vi "Get Devs and Channels.vi"(8 "error in (no error)":errorcluster, 11 "Simulated Sequencer in":refnum<class "Simulated Sequencer.lvclass">) -> (0 "error out":errorcluster, 3 "Simulated Sequencer out":refnum<class "Simulated Sequencer.lvclass">)   [LabVIEW 2015, in "Simulated Sequencer.lvlib" / "Simulated Sequencer.lvclass"]
uses:
  Simulated Sequencer.lvclass
  Sequencer/Sequencer/Daq Channel Info.ctl
  Sequencer/Sequencer/Sequencer.lvclass
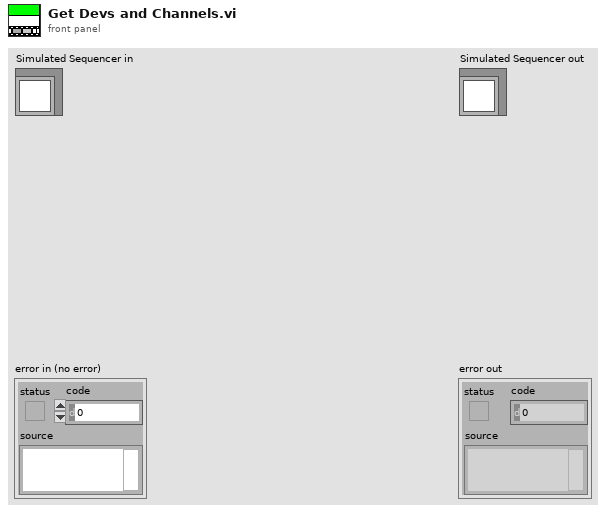
[diagram p1: front panel]
types:
  T1 = typedef "Sequencer.lvlib/Sequencer.lvclass/Daq Channel Info.ctl" = cluster{"DevNames":tag[], "AO.PhysicalChans":tag[][], "DO.Lines":tag[][], "AI.PhysicalChans":tag[][]}
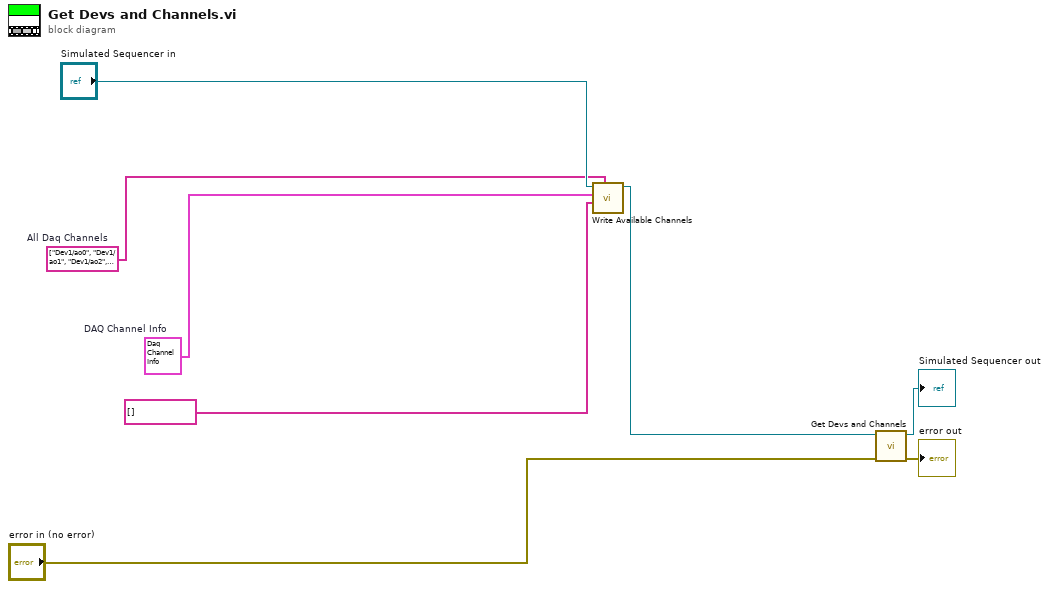
[diagram p0: block diagram]
diagram:
  w1 = tag[] ["Dev1/ao0", "Dev1/ao1", "Dev1/ao2", "Dev1/ao3", "", ""]  # All Daq Channels
  w3 = T1 {"DevNames"=["Dev1", "Dev2"], "AO.PhysicalChans"=[["Dev1/ao0", "Dev1/ao1", "Dev1/ao2", "Dev1/ao3"], ["Dev2/ao0", "Dev2/ao1", "Dev2/ao2", "Dev2/ao3"]], "DO.Lines"=[["Dev1/port0/line0", "Dev1/port0/line1", "Dev1/port0/line2", "Dev1/port0/line3", "Dev1/port0/line4", "Dev1/port0/line5", "Dev1/port0/line6", "Dev1/port0/line7", "Dev1/port0/line8", "Dev1/port0/line9", "Dev1/port0/line10", "Dev1/port0/line11", "Dev1/port0/line12", "Dev1/port0/line13", "Dev1/port0/line14", "Dev1/port0/line15", "Dev1/port0/line16", "Dev1/port0/line17", "Dev1/port0/line18", "Dev1/port0/line19", "Dev1/port0/line20", "Dev1/port0/line21", "Dev1/port0/line22", "Dev1/port0/line23", "Dev1/port0/line24", "Dev1/port0/line25", "Dev1/port0/line26", "Dev1/port0/line27", "Dev1/port0/line28", "Dev1/port0/line29", "Dev1/port0/line30", "Dev1/port0/line31", "Dev1/port1/line0", "Dev1/port1/line1", "Dev1/port1/line2", "Dev1/port1/line3", "Dev1/port1/line4", "Dev1/port1/line5", "Dev1/port1/line6", "Dev1/port1/line7", "Dev1/port2/line0", "Dev1/port2/line1", "Dev1/port2/line2", "Dev1/port2/line3", "Dev1/port2/line4", "Dev1/port2/line5", "Dev1/port2/line6", "Dev1/port2/line7"], ["Dev2/port0/line0", "Dev2/port0/line1", "Dev2/port0/line2", "Dev2/port0/line3", "Dev2/port0/line4", "Dev2/port0/line5", "Dev2/port0/line6", "Dev2/port0/line7", "Dev2/port0/line8", "Dev2/port0/line9", "Dev2/port0/line10", "Dev2/port0/line11", "Dev2/port0/line12", "Dev2/port0/line13", "Dev2/port0/line14", "Dev2/port0/line15", "Dev2/port0/line16", "Dev2/port0/line17", "Dev2/port0/line18", "Dev2/port0/line19", "Dev2/port0/line20", "Dev2/port0/line21", "Dev2/port0/line22", "Dev2/port0/line23", "Dev2/port0/line24", "Dev2/port0/line25", "Dev2/port0/line26", "Dev2/port0/line27", "Dev2/port0/line28", "Dev2/port0/line29", "Dev2/port0/line30", "Dev2/port0/line31", "Dev2/port1/line0", "Dev2/port1/line1", "Dev2/port1/line2", "Dev2/port1/line3", "Dev2/port1/line4", "Dev2/port1/line5", "Dev2/port1/line6", "Dev2/port1/line7", "Dev2/port2/line0", "Dev2/port2/line1", "Dev2/port2/line2", "Dev2/port2/line3", "Dev2/port2/line4", "Dev2/port2/line5", "Dev2/port2/line6", "Dev2/port2/line7"]], "AI.PhysicalChans"=[["Dev1/ai0", "Dev1/ai1", "Dev1/ai2", "Dev1/ai3", "Dev1/ai4", "Dev1/ai5", "Dev1/ai6", "Dev1/ai7", "Dev1/ai8", "Dev1/ai9", "Dev1/ai10", "Dev1/ai11", "Dev1/ai12", "Dev1/ai13", "Dev1/ai14", "Dev1/ai15", "Dev1/ai16", "Dev1/ai17", "Dev1/ai18", "Dev1/ai19", "Dev1/ai20", "Dev1/ai21", "Dev1/ai22", "Dev1/ai23", "Dev1/ai24", "Dev1/ai25", "Dev1/ai26", "Dev1/ai27", "Dev1/ai28", "Dev1/ai29", "Dev1/ai30", "Dev1/ai31"], ["Dev2/ai0", "Dev2/ai1", "Dev2/ai2", "Dev2/ai3", "Dev2/ai4", "Dev2/ai5", "Dev2/ai6", "Dev2/ai7", "Dev2/ai8", "Dev2/ai9", "Dev2/ai10", "Dev2/ai11", "Dev2/ai12", "Dev2/ai13", "Dev2/ai14", "Dev2/ai15", "Dev2/ai16", "Dev2/ai17", "Dev2/ai18", "Dev2/ai19", "Dev2/ai20", "Dev2/ai21", "Dev2/ai22", "Dev2/ai23", "Dev2/ai24", "Dev2/ai25", "Dev2/ai26", "Dev2/ai27", "Dev2/ai28", "Dev2/ai29", "Dev2/ai30", "Dev2/ai31"]]}  # DAQ Channel Info
  n1 = call "Write Available Channels.vi"("All Daq Channels"=w1, "Used DAQChannels"=tag[] [], "DAQ Channel Info"=w3, "Sequencer in"="Simulated Sequencer in") -> ("Sequencer out"=w4:refnum<class "Simulated Sequencer.lvclass">)  [unwired: 6 in, 1 out]
  n2 = call-parent "Get Devs and Channels.vi"("error in (no error)"="error in (no error)", "Sequencer in"=w4) -> ("error out"=→"error out":errorcluster, "Sequencer out"=→"Simulated Sequencer out":refnum<class "Simulated Sequencer.lvclass">)  [unwired: 8 in]
